vi "Pickering 4 wire-3VoltageAmps.vi"(0 "26":string[](array[combo])=["y6", "NC"], 1 "27":string[](array[combo])=["y8", "NC"], 2 "28":string[](array[combo])=["y1", "NC"], 3 "1":string[](array[combo])=["y3", "NC"], 8 "5":string[](array[combo])=["y4", "NC"], 9 "4":string[](array[combo])=["y5", "NC"], 10 "3":string[](array[combo])=["NC", "NC"], 11 "2":string[](array[combo])=["y7", "NC"]) -> ()   [LabVIEW 2011]
uses:
  Lockin/source/subVI/Lock-in Globles.vi
panel:
  in  "Initialize":bool
  in  "Pickering status":path=path "C:/LabView/PPMS basic VIs/Switch Status.txt"
  in  "Disconnect all?":bool
  in  "IVI Option String":string="Simulate=0,RangeCheck=1,QueryInstrStatus=0,Cache=1,DriverSetup=Model:40-726-511-M;"
  in  "VISA Resource Name":string="PXI9::13::INSTR"
  in  "X Channel Ground":string="x9"
  in  "Discharge Y Channels?":bool=TRUE
  in  "Discharge X channels?":bool=TRUE
  in  "Y Channel Ground":string="y1"
  # "4 wire              measurements\nFeature:\n1, Multiple connections\n2, Make before break\n3, First run resets device\n\nNotes:\nLock-in 1: I+/I- -->AO0/AI0, board 0\n\nLock-in 3: V+/V-  --> AI0, board 1.  \n  V+/V- conencted to y3 and y4. OSC output should set the same as Lock-in 1\n\nLock-in 2: I2+/I2- -->AO1/AI1, board 0\n\nLock-in 4: V2+/V2- -> y7/y8"
  # "5"
  # "4"
  # "3"
  # "2"
  # "26"
  # "27"
  # "28"
  # "1"
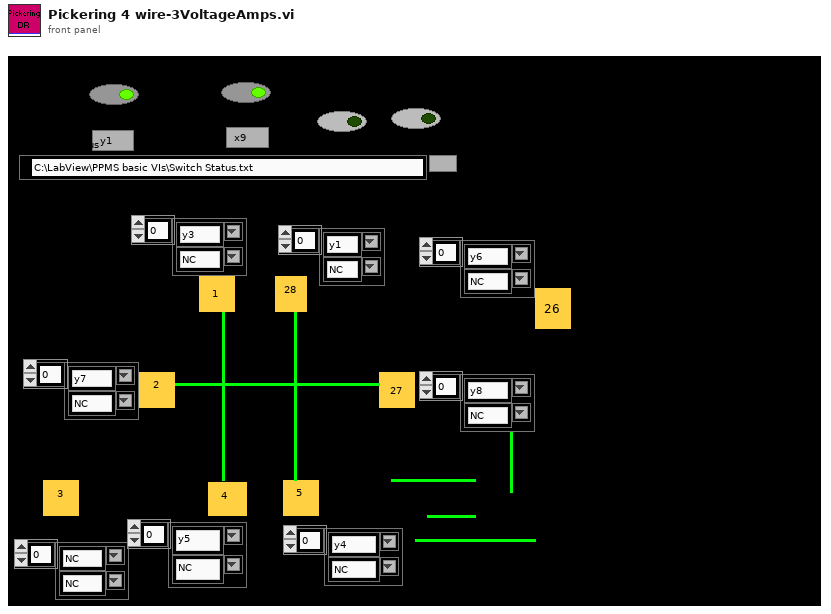
[diagram p1: front panel]
types:
  T1 = cluster{"output string":string, "output string":string}
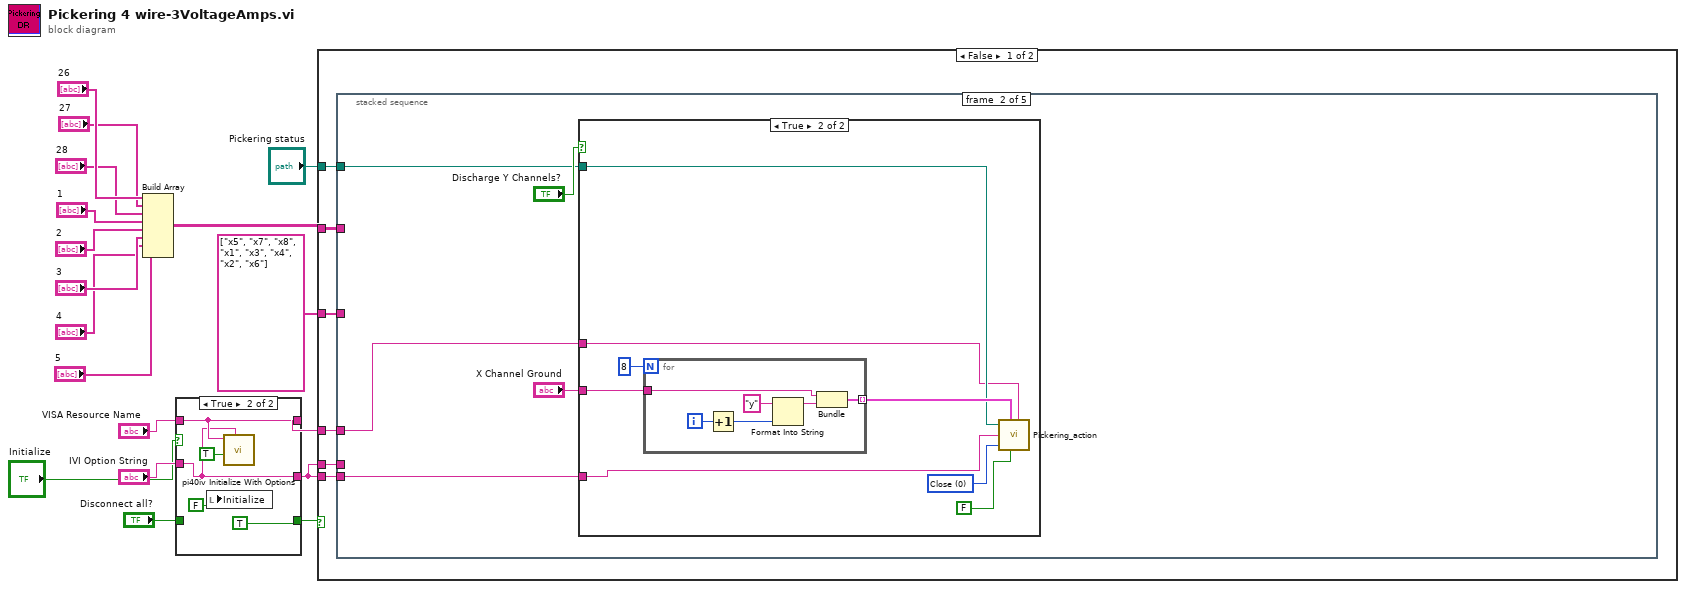
[diagram p0: block diagram]
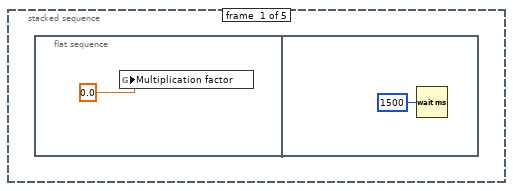
[diagram p3: hidden frame]
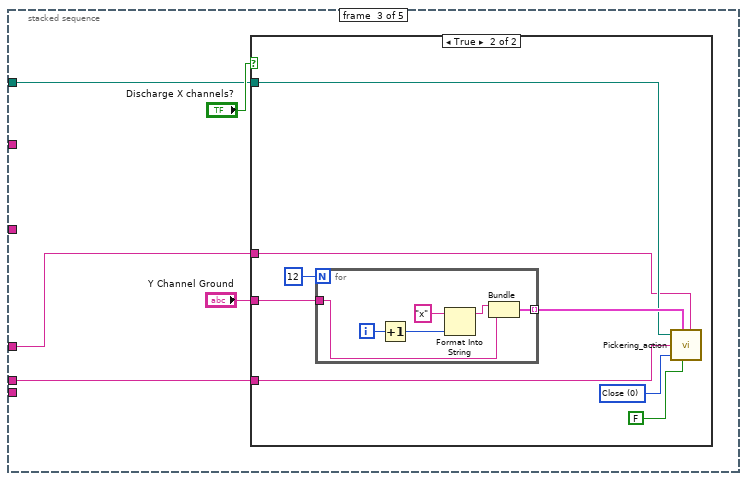
[diagram p5: hidden frame]
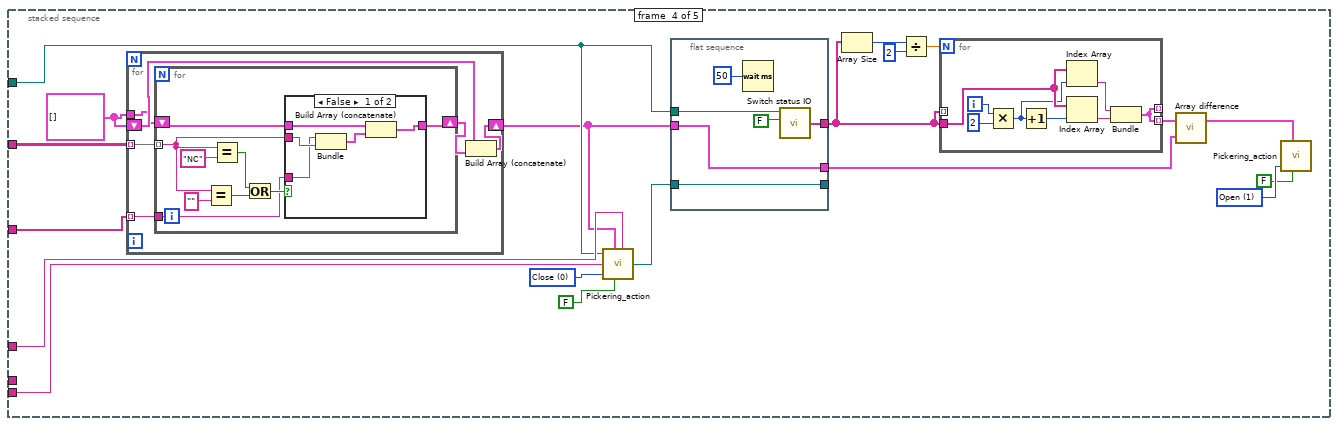
[diagram p7: hidden frame]
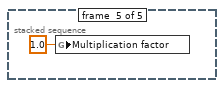
[diagram p9: hidden frame]
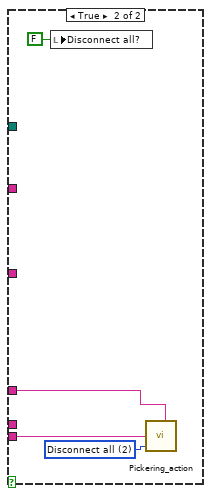
[diagram p10: hidden frame]
diagram:
  n1 = Build Array("26", "27", "28", "1", "2", "3", "4", "5") -> (w8:string[][])
  n2 = case shown="True" "Initialize" {
    tunnel: "VISA Resource Name" -> [w21 w26]
    tunnel: [w21 w26] -> w6
    tunnel: "IVI Option String" -> [w20 w25]
    tunnel: [w20 w25] -> w4
    tunnel: "Disconnect all?" -> [w19 _]
    tunnel: [w19 TRUE ("reset device")] -> w1
    frame False {
    }
    frame True {
      n3 = local write "Initialize"(FALSE ("reset device")) -> ()
      n4 = call <instrlib>:"pi40iv Initialize With Options.vi"("option string"=w25, "reset device"=TRUE, "resource name"=w26) -> ()  [unwired: 7 in, 2 out]
    }
  }
  n5 = case shown="False" w1 {
    tunnel: w8 -> [w32 _]
    tunnel: string[] ["x5", "x7", "x8", "x1", "x3", "x4", "x2", "x6"] -> [w31 _]
    tunnel: w4 -> [w30 w129]
    tunnel: w6 -> [w29 w128]
    tunnel: "Pickering status" -> [w28 _]
    tunnel: w4 -> [w27 _]
    frame False {
      n6 = stacked-sequence {
        tunnel: w32 -> [_ _ _ w91 _]
        tunnel: w31 -> [_ _ _ w90 _]
        tunnel: w30 -> [_ w37 _ w89 _]
        tunnel: w29 -> [_ w35 w55 w88 _]
        tunnel: w28 -> [_ w36 w56 w87 _]
        tunnel: w27 -> [_ _ w54 _ _]
        frame #0 {
          n7 = flat-sequence {
            frame #0 {
              n8 = global write "Lock-in Globles.vi" "Multiplication factor"(0.0 ("Multiplication factor")) -> ()
            }
            frame #1 {
              n9 = Wait (ms)(milliseconds to wait=u32 1500) -> ()  [unwired: 1 out]
            }
          }
        }
        frame #1 {
          n10 = case shown="True" "Discharge Y Channels?" {
            tunnel: "X Channel Ground" -> [_ w47]
            tunnel: w37 -> [_ w43]
            tunnel: w35 -> [_ w40]
            tunnel: w36 -> [_ w42]
            frame False {
            }
            frame True {
              w44 = u16 0 items=["Close", "Open", "Disconnect all"] ("Action")
              n11 = for {
                N: 8 -> [_]
                tunnel: w47 -> [w49]
                tunnel: [w48] -> w45 mode=indexing
                i -> [w52]
                n12 = Increment(x=w52) -> (x+1=w51:i32)
                n13 = Format Into String(initial string="y", w51) -> (resulting string=w50:string)  [unwired: 2 in, 1 out]
                n14 = Bundle("X Channel Ground"=w49, w50) -> (w48:cluster{"X Channel Ground":string, string})  [unwired: 1 in]
              }
              n15 = call "Pickering_action.vi"("Pickering status"=w42, "Array"=w45, "option string"=w43, "Action"=w44, "Initialize"=FALSE, "resource name"=w40) -> ()  [unwired: 3 in, 1 out]
            }
          }
        }
        frame #2 {
          n16 = case shown="True" "Discharge X channels?" {
            tunnel: "Y Channel Ground" -> [_ w66]
            tunnel: w56 -> [_ w63]
            tunnel: w55 -> [_ w62]
            tunnel: w54 -> [_ w61]
            frame False {
            }
            frame True {
              w59 = u16 0 items=["Close", "Open", "Disconnect all"] ("Action")
              n17 = for {
                N: 12 -> [_]
                tunnel: w66 -> [w67]
                tunnel: [w69] -> w64 mode=indexing
                i -> [w71]
                n18 = Increment(x=w71) -> (x+1=w70:i32)
                n19 = Format Into String(initial string="x", w70) -> (resulting string=w68:string)  [unwired: 2 in, 1 out]
                n20 = Bundle(w68, "Y Channel Ground"=w67) -> (w69:cluster{string, "Y Channel Ground":string})  [unwired: 1 in]
              }
              n21 = call "Pickering_action.vi"("Pickering status"=w63, "Array"=w64, "option string"=w61, "Action"=w59, "Initialize"=FALSE, "resource name"=w62) -> ()  [unwired: 3 in, 1 out]
            }
          }
        }
        frame #3 {
          w78 = u16 1 items=["Close", "Open", "Disconnect all"] ("Action")
          w86 = u16 0 items=["Close", "Open", "Disconnect all"] ("Action")
          w82 = cluster{"5":string, string}[] []
          n22 = for {
            tunnel: w91 -> [w110] mode=indexing
            tunnel: w90 -> [w111] mode=indexing
            shift-right: [w109] -> w83
            shift-left: w82 -> [w107]
            tunnel: w82 -> [w106]
            n23 = for {
              tunnel: w111 -> [w115]
              tunnel: w110 -> [w114] mode=indexing
              shift-right: [w112] -> w108
              shift-left: w106 -> [w113]
              n24 = Equal?(x=w114, y="") -> (x = y?=w117:bool)
              n25 = Equal?(x=w114, y="NC") -> (x = y?=w119:bool)
              n26 = Or(x=w119, y=w117) -> (x .or. y?=w118:bool)
              n27 = case shown="False" w118 {
                tunnel: w115 -> [w121 _]
                tunnel: w114 -> [w122 _]
                tunnel: [w124 w126] -> w112
                tunnel: w113 -> [w123 w126]
                frame False {
                  n28 = Bundle(w121, "26"=w122) -> (w125:cluster{string, "26":string})  [unwired: 1 in]
                  n29 = Build Array (concatenate)(w123, w125) -> (w124:cluster{"5":string, "26":string}[])
                }
                frame True {
                }
              }
            }
            n30 = Build Array (concatenate)(w107, w108) -> (w109:cluster{"5":string, string}[])
          }
          n31 = call "Pickering_action.vi"("Pickering status"=w87, "Array"=w83, "option string"=w89, "Action"=w86, "Initialize"=FALSE, "resource name"=w88) -> ("instrument handle out"=w84:refnum<k15>)  [unwired: 3 in]
          n32 = flat-sequence {
            tunnel: w84 -> [w104]
            tunnel: [w104] -> _
            tunnel: [w103] -> w77
            tunnel: w87 -> [w102]
            tunnel: w83 -> [w100]
            tunnel: [w100] -> w75
            frame #0 {
              n33 = Wait (ms)(milliseconds to wait=u32 50) -> ()  [unwired: 1 out]
              n34 = call "Switch status IO.vi"("Write: T\nRead: F"=FALSE ("Write: T\nRead: F"), "Path"=w102) -> ("String out"=w103:string[])  [unwired: 4 in]
            }
          }
          n35 = Array Size(array=w77) -> (size(s)=w81:i32)
          n36 = Divide(x=w81, y=2) -> (x/y=w79:dbl)
          n37 = for {
            N: w79 -> [_]
            tunnel: w77 -> [w99]
            tunnel: w77 -> [_] mode=indexing
            tunnel: [w92] -> _ mode=indexing
            tunnel: [w92] -> w76 mode=indexing
            i -> [w95]
            n38 = Multiply(x=w95, y=2) -> (x*y=w93:i32)
            n39 = Increment(x=w93) -> (x+1=w98:i32)
            n40 = Index Array(array=w99, index=w93) -> (element=w97:string)
            n41 = Index Array(array=w99, index=w98) -> (element=w96:string)
            n42 = Bundle("output string"=w97, "output string"=w96) -> (w92:T1)  [unwired: 1 in]
          }
          n43 = call "Array difference.vi"("Array 2"=w75, "Array 1"=w76) -> ("Array 1-(array1&2)"=w74:cluster{"String":string, "String 2":string}[])  [unwired: 1 out]
          n44 = call "Pickering_action.vi"("Array"=w74, "Action"=w78, "Initialize"=FALSE) -> ()  [unwired: 6 in, 1 out]
        }
        frame #4 {
          n45 = global write "Lock-in Globles.vi" "Multiplication factor"(1.0 ("Multiplication factor")) -> ()
        }
      }
    }
    frame True {
      w130 = u16 2 items=["Close", "Open", "Disconnect all"] ("Action")
      n46 = local write "Disconnect all?"(FALSE ("Disconnect all?")) -> ()
      n47 = call "Pickering_action.vi"("option string"=w129, "Action"=w130, "resource name"=w128) -> ()  [unwired: 6 in, 1 out]
    }
  }
